vi "007 Gràfic temperatures i alarmes.vi"() -> ()   [LabVIEW 2019]
panel:
  out "Min Temp":dbl
  out "Max Temp":dbl
  out "Alarma límit inf":bool
  out "Alarma límit sup":bool
  in  "Limit inferior":dbl
  in  "Limit superior":dbl
  out "Waveform Chart":T1(graph)
  out "Data":dbl
  in  "Conf. temperatura":T2
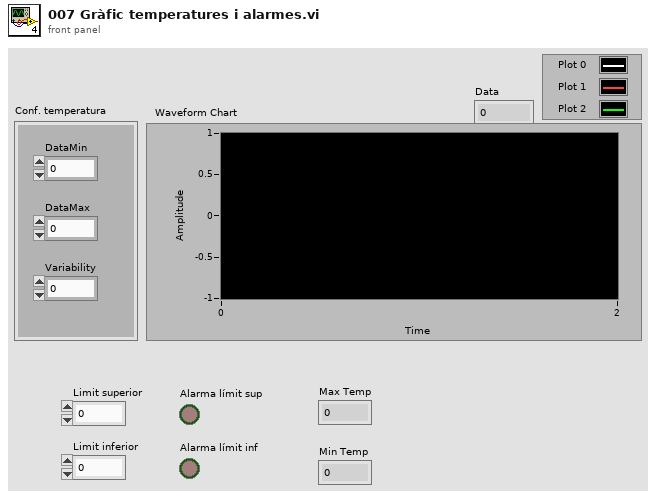
[diagram p1: front panel]
types:
  T1 = cluster{"Limit inferior":dbl, "Data":dbl, "Limit superior":dbl}
  T2 = cluster{"DataMin":dbl, "DataMax":dbl, "Variability":dbl}
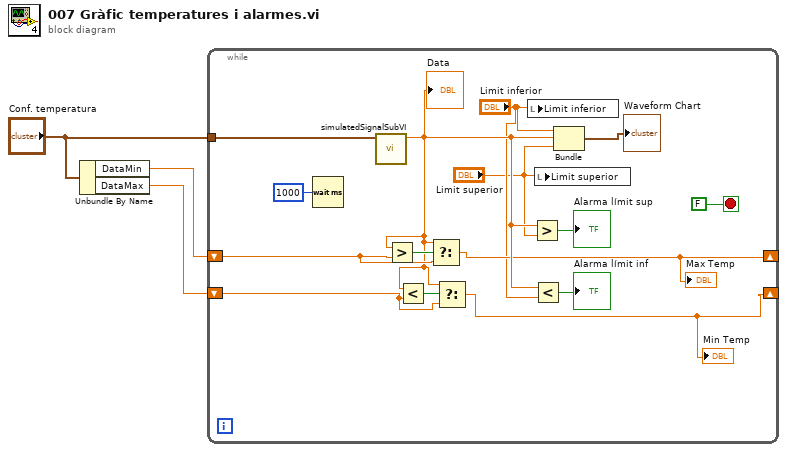
[diagram p0: block diagram]
diagram:
  n1 = Unbundle By Name("Conf. temperatura") -> ("DataMin"=w2:dbl, "DataMax"=w1:dbl)
  n2 = while {
    shift-right: [w7] -> _
    shift-left: w2 -> [w12]
    shift-right: [w8] -> _
    shift-left: w1 -> [w9]
    tunnel: "Conf. temperatura" -> [w4]
    stop <- FALSE stop-if-true
    n3 = Wait (ms)(milliseconds to wait=u32 1000) -> ()  [unwired: 1 out]
    n4 = call "simulatedSignalSubVI.vi"("Channel"=w4) -> ("Data"=w10:dbl)  [unwired: 10 in]
    "Data" <- w10
    n5 = Greater?(x=w10, y=w12) -> (0:w13:bool)
    n6 = Less?(x=w10, y=w9) -> (x < y?=w11:bool)
    n7 = Select(t=w10, s=w13, f=w12) -> (s? t:f=w7:dbl)
    "Max Temp" <- w7
    n8 = Select(t=w10, s=w11, f=w9) -> (s? t:f=w8:dbl)
    "Min Temp" <- w8
    n9 = local write "Limit inferior"("Limit inferior") -> ()
    n10 = Greater?(x=w10, y="Limit superior") -> (0:→"Alarma límit sup":bool)
    n11 = Less?(x=w10, y="Limit inferior") -> (x < y?=→"Alarma límit inf":bool)
    n12 = local write "Limit superior"("Limit superior") -> ()
    n13 = Bundle("Limit inferior"="Limit inferior", "Data"=w10, "Limit superior"="Limit superior") -> (→"Waveform Chart":T1)  [unwired: 1 in]
  }
